vi "Forward Kinematics.vi"(8 "Radii (ft)":T2 {"Right Back radius" format="%.2f"; "Right Front radius" format="%.2f"; "Left Back radius" format="%.2f"; "Left Front radius" format="%.2f"}, 10 "Steer Angles (degrees)":T1, 11 "Drive Velocities (ft/s)":T1) -> (3 "Robot Velocities (ft and deg)/s":cluster{"vx":dbl, "vy":dbl, "w":dbl})   [LabVIEW 2020]
uses:
  <vilib>/Analysis/NI_AALPro.lvlib
  <vilib>/Analysis/NI_AALBase.lvlib
  <vilib>/Analysis/baseanly.llb/A x Vector.vi
  <vilib>/Analysis/_algsub.llb/Real PseudoInverse Matrix.vi
  ctl/Radii.ctl
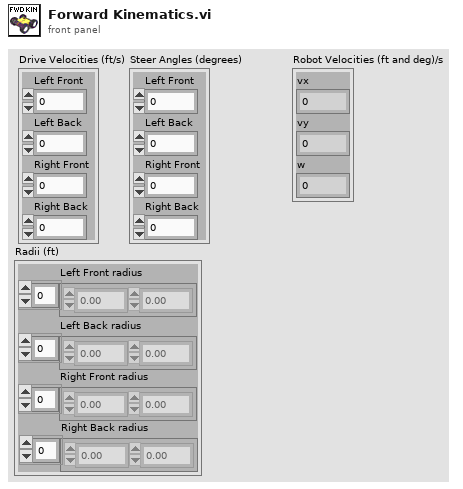
[diagram p1: front panel]
types:
  T1 = cluster{"Left Front":i32, "Left Back":i32, "Right Front":i32, "Right Back":i32}
  T2 = typedef "Radii.ctl" = cluster{"Left Front radius":dbl[], "Left Back radius":dbl[], "Right Front radius":dbl[], "Right Back radius":dbl[]}
  T3 = typedef "NI_Matrix.lvlib/RealMatrix.ctl" = dbl[][]
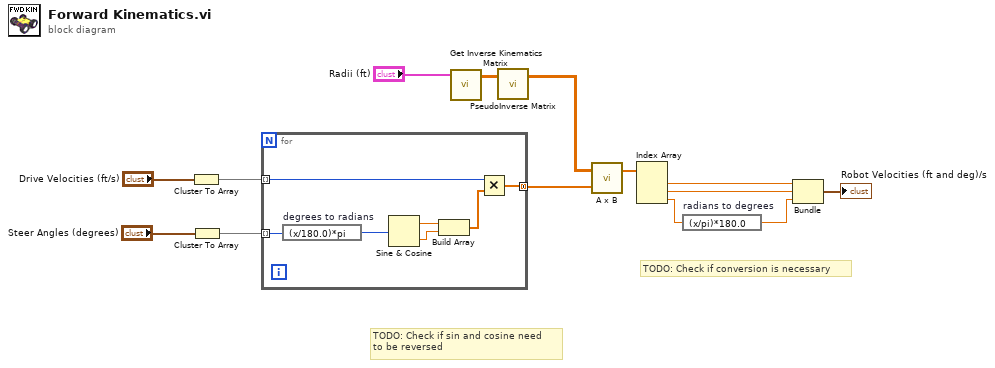
[diagram p0: block diagram]
diagram:
  # "TODO: Check if sin and cosine need\nto be reversed"
  # "TODO: Check if conversion is necessary"
  n1 = Cluster To Array(cluster="Drive Velocities (ft/s)") -> (array=w10:i32[])
  n2 = Cluster To Array(cluster="Steer Angles (degrees)") -> (array=w9:i32[])
  n3 = for {
    tunnel: w10 -> [w17] mode=indexing
    tunnel: w9 -> [w21] mode=indexing
    tunnel: [w15] -> w8 mode=concatenating
    n4 = expression code="(x/180.0)*pi" "degrees to radians"(w21) -> (w20:i32)
    n5 = Sine & Cosine(0:w20) -> (1:w19:dbl, 2:w18:dbl)
    n6 = Build Array(w19, w18) -> (w16:dbl[])
    n7 = Multiply(x=w17, y=w16) -> (x*y=w15:dbl[])
  }
  n8 = call "Get Inverse Kinematics Matrix.vi"("Radii (ft)"="Radii (ft)") -> ("Real Matrix"=w13:T3)  [unwired: 10 in]
  n9 = call-poly <vilib>:"PseudoInverse Matrix.vi"("Input Matrix"=w13) -> ("PseudoInverse Matrix"=w7:T3)  [unwired: 1 in, 1 out]
  n10 = call-poly <vilib>:"A x B.vi"("Vector"=w8, "A"=w7) -> ("A x Vector"=w6:dbl[])  [unwired: 1 out]
  n11 = Index Array(array=w6) -> (element #1=w5:dbl, element #2=w4:dbl, element #3=w3:dbl)  [unwired: 3 in]
  n12 = expression code="(x/pi)*180.0" "radians to degrees"(w3) -> (w2:dbl)
  n13 = Bundle(w5, w4, w2) -> (→"Robot Velocities (ft and deg)/s":cluster{dbl, dbl, dbl})  [unwired: 1 in]
